vi "Sample In.vi"(8 "error in (no error)":errorcluster, 10 "Sample":refnum<class "Sample.lvclass">, 11 "CO2 Actor in":refnum<class "CO2 Actor.lvclass">) -> (0 "error out":errorcluster, 3 "CO2 Actor out":refnum<class "CO2 Actor.lvclass">)   [LabVIEW 2015, in "cRIO-Carbondioxide.lvlib" / "CO2-Actor.lvlib" / "CO2 Actor.lvclass"]
uses:
  CO2 Actor.lvclass
  subs/Sample/Sample.lvclass
  <vilib>/ActorFramework/Actor/Actor.lvclass/Actor.ctl
  <vilib>/ActorFramework/Message Enqueuer/Message Enqueuer.lvclass/Message Enqueuer.ctl
  <vilib>/ActorFramework/Actor/Read Self Enqueuer.vi
  <vilib>/ActorFramework/Message Enqueuer/Init from Existing Queue.vi
  <vilib>/ActorFramework/Actor/Actor.lvclass
  <vilib>/ActorFramework/Message Enqueuer/Message Enqueuer.lvclass
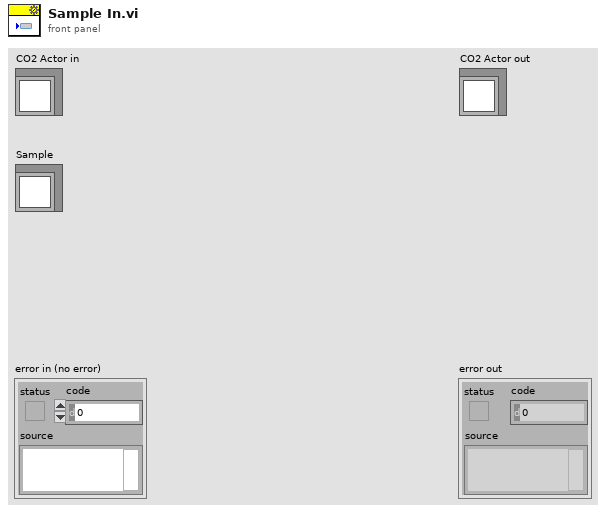
[diagram p1: front panel]
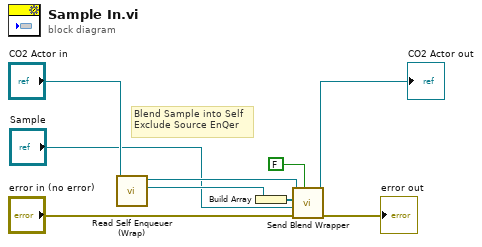
[diagram p0: block diagram]
diagram:
  # "Blend Sample into Self\nExclude Source EnQer"
  n1 = call "Read Self Enqueuer (Wrap).vi"("CO2 Actor in"="CO2 Actor in") -> ("Actor Framework:Message Enqueuer"=w9:refnum<class "Message Enqueuer.lvclass">, "CO2 Actor out"=w7:refnum<class "CO2 Actor.lvclass">)  [unwired: 9 in]
  n2 = Build Array(w9) -> (w8:refnum<class "Message Enqueuer.lvclass">[])
  n3 = call-dynamic "Send Blend Wrapper.vi"("Include Source EnQr (T)"=FALSE, "error in (no error)"="error in (no error)", "Sample to Blend"="Sample", "Send to"=w8, "CO2 Actor in"=w7) -> ("error out"=→"error out":errorcluster, "CO2 Actor out"=→"CO2 Actor out":refnum<class "CO2 Actor.lvclass">)  [unwired: 5 in]
